vi "Generate Hardware Fingerprint.vi"(11 "Product ID":string) -> (3 "Hash":string)   [LabVIEW 2012]
doc: "This VI generates a hardware fingerprint for validating software installs. The hash, the final output, should be unique for different hardware setups. However, the presence ofa <b>Product ID</b> allows us to ensure that even on the same setup, we can produce a unique hash for two different installs. Or ensure that a file might be specifically intended for a particular setup."
panel:
  out "Encrypt":string
  # "The value under Panel ID will b written to the configuration file so that the file itself will be keyed to the device.  This value can be any string.  IN addition, the hash should be written to the configuration file so that we don't have to have the user enter it every time."
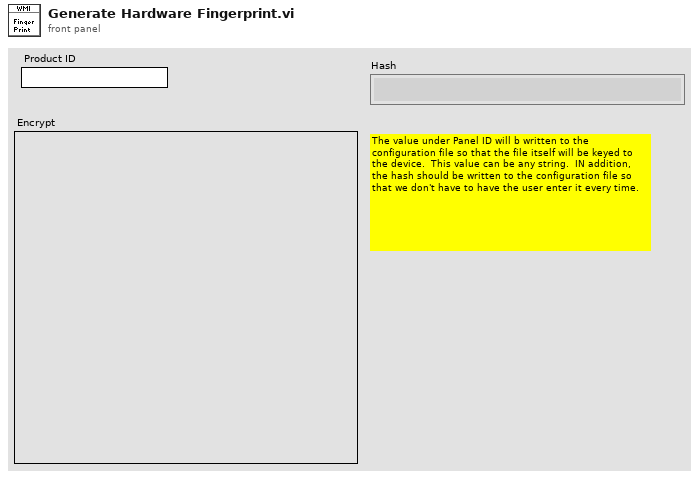
[diagram p1: front panel]
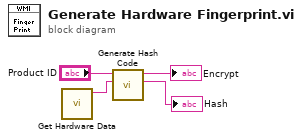
[diagram p0: block diagram]
diagram:
  n1 = call "Get Hardware Data.vi"() -> ("Fingerprint"=w3:string)  [unwired: 11 in]
  n2 = call "Generate Hash Code.vi"("Fingerprint"=w3, "Product ID"="Product ID") -> ("Hash"=→"Hash":string, "Encrypt"=→"Encrypt":string)  [unwired: 8 in]
